vi "Main.vi"(11 "Module Admin":refnum<class "Delacor_lib_QMH_Module Admin.lvclass">) -> ()   [LabVIEW 2020, in "SimpleDependencyInspector.lvlib"]
doc: "This template is based off of the Queued Message Handler design pattern and the Queued Message Handler project template that ships with LabVIEW.\n\nThe main difference is that the queue is private to this module and communication between modules is performed via Broadcast and Request events.\n\nRequest events are wrapped in public API methods and are handled in the Event Handling Loop (EHL) of this VI. Any module can register for Broadcast events sent by this module. The EHL generates messages based on user interface actions.\n\nThe Message Handling Loop (MHL) processes messages generated by the EHL, or by other messages. The messages are string values, so new messages can be added easily to the Message Cases case structure in the MHL. Each message cluster can also provide an optional value for Message Data, which is a variant that can be converted to whatever message-specific data is required.\n_____\nBased on DQMH Project Template 7.0.1.1316.\n\n<b>Note:</b> This VI was modified by the <b>Validate DQMH Module</b> tool to wrap the FP.Open method in the module close code with a Conditional Disable Structure so it does not execute when the Main VI is running as a built EXE."
uses:
  SimpleDependencyInspector.lvlib
  <vilib>/Delacor/Delacor QMH/Libraries/Module Admin_class/Delacor_lib_QMH_Module Admin.lvclass
  Module Data--cluster.ctl
  <vilib>/Delacor/Delacor QMH/Libraries/Message Queue_class/Delacor_lib_QMH_Message Queue.lvclass/Delacor_lib_QMH_Message Queue.ctl
  Stop Argument--cluster.ctl
  Inspect Project Dependencies Argument--cluster.ctl
  Image Type--enum.ctl
  <vilib>/Delacor/Delacor QMH/Libraries/Module Admin_class/Delacor_lib_QMH_Module Admin.lvclass/Delacor_lib_QMH_Module Admin.ctl
  <vilib>/Delacor/Delacor QMH/Libraries/Message Queue_class/Delacor_lib_QMH_Enqueue Message (Single).vi
  <vilib>/Delacor/Delacor QMH/Libraries/Module Admin_class/Delacor_lib_QMH_Get External Launch.vi
  <vilib>/Delacor/Delacor QMH/Libraries/Message Queue_class/Delacor_lib_QMH_Message Queue.lvclass
panel:
  out "Dependencies Plot":picture
  out "error out":errorcluster
  out "Status":string
  in  "Home":bool
  in  "About":bool
  in  "Zoom In":bool
  in  "Zoom Out":bool
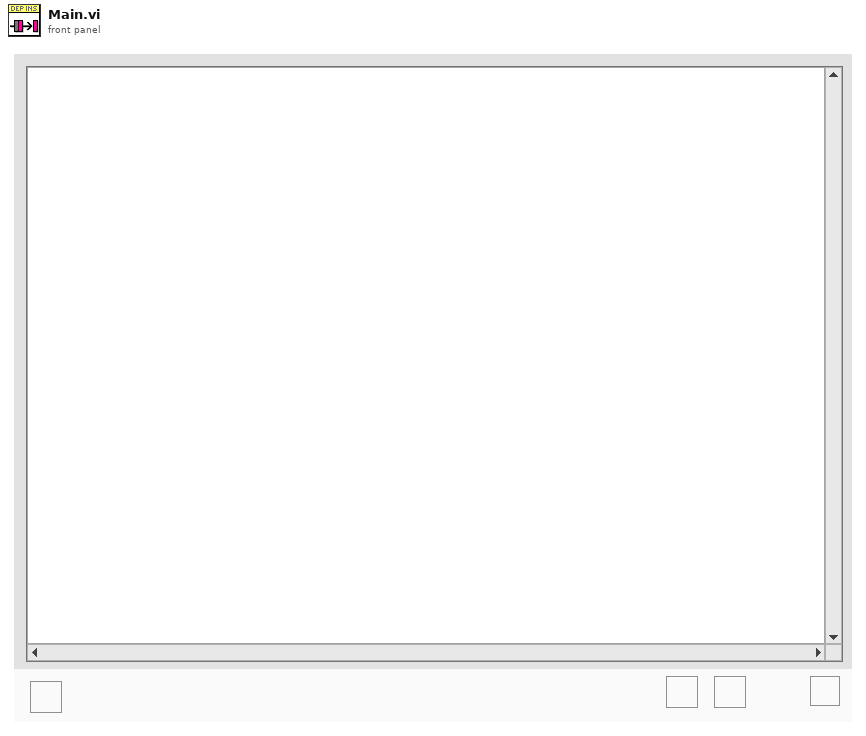
[diagram p1: front panel]
types:
  T1 = typedef "SimpleDependencyInspector.lvlib/Request Events--cluster.ctl" = cluster{"Stop Module":refnum<user-event>, "Show Panel":refnum<user-event>, "Hide Panel":refnum<user-event>, "Get Module Execution Status":refnum<user-event>, "Show Diagram":refnum<user-event>, "Inspect Project Dependencies":refnum<user-event>, "Private":cluster{"Wake Up HL":refnum<user-event>}}
  T2 = typedef "SimpleDependencyInspector.lvlib/Module Data--cluster.ctl" = cluster{"Status":string}
  T3 = enum32{"invalid lock state", "Not Locked", "Locked (No Password)", "Password-protected"}
  T4 = typedef "SimpleDependencyInspector.lvlib/Stop Argument--cluster.ctl" = cluster{"Origin":string, "Exit via Stop Module Req?":bool, "Wait for Module to stop?":bool}
  T5 = typedef "SimpleDependencyInspector.lvlib/Inspect Project Dependencies Argument--cluster.ctl" = cluster{"Path(s) Selection":path[], "Include vi.lib":bool, "pattern Search":string[], "pattern To include in Plot":string[], "Working Path":path, "Img Type":T6}
  T6 = typedef "SimpleDependencyInspector.lvlib/Image Type--enum.ctl" = enum16{"JPEG", "PNG", "BMP", "SVG"}
  T7 = enum32{"Invalid", "Standard", "Closed", "Hidden", "Minimized", "Maximized"}
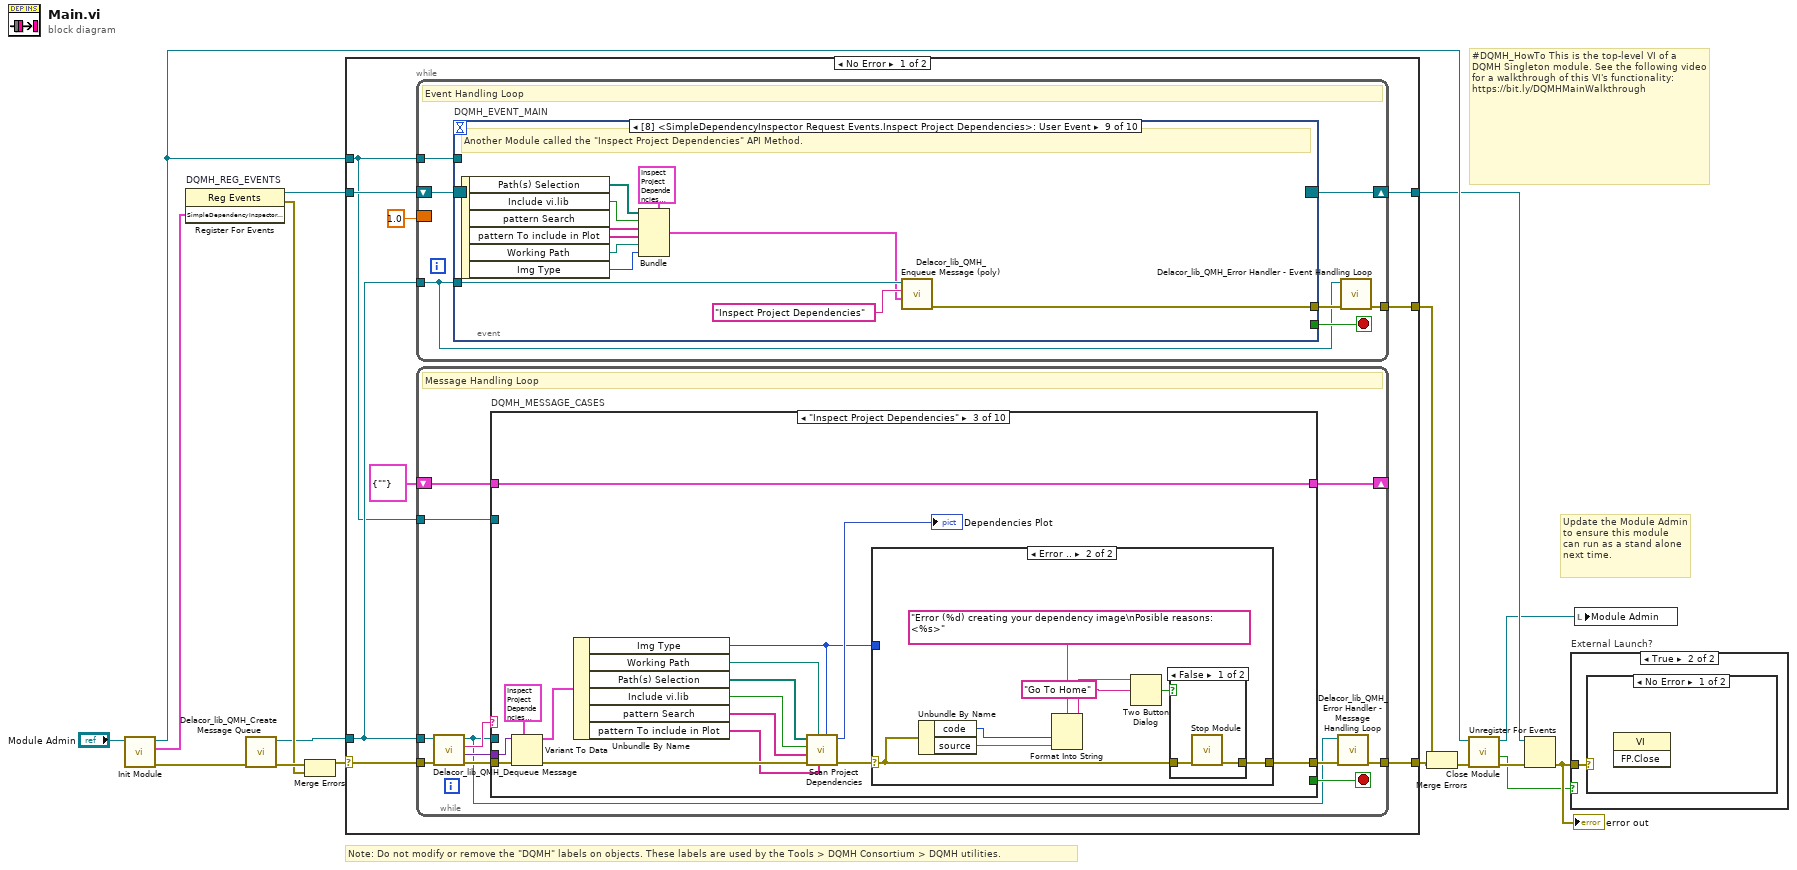
[diagram p0: block diagram]
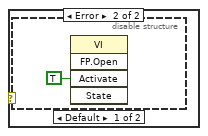
[diagram p3: hidden frame]
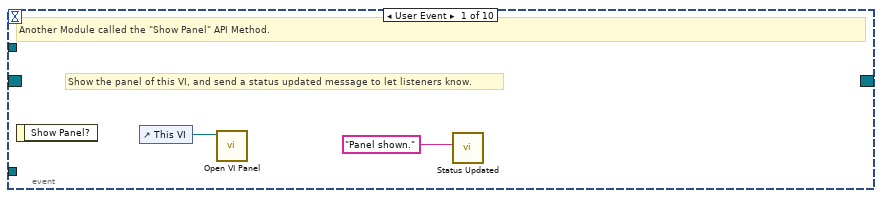
[diagram p5: hidden frame]
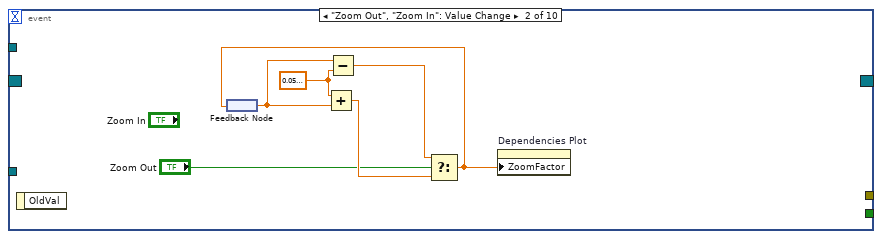
[diagram p6: hidden frame]
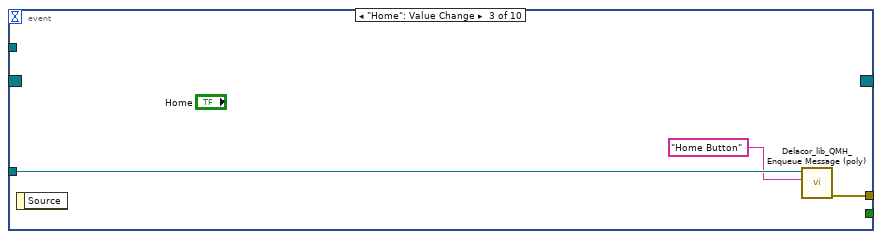
[diagram p7: hidden frame]
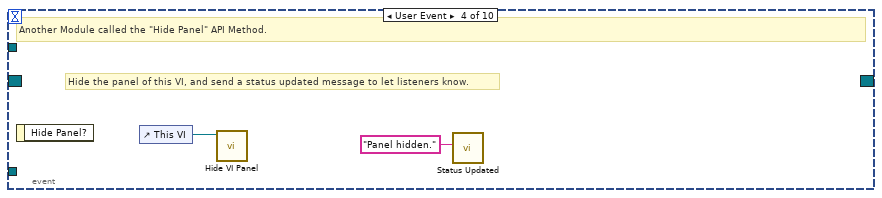
[diagram p8: hidden frame]
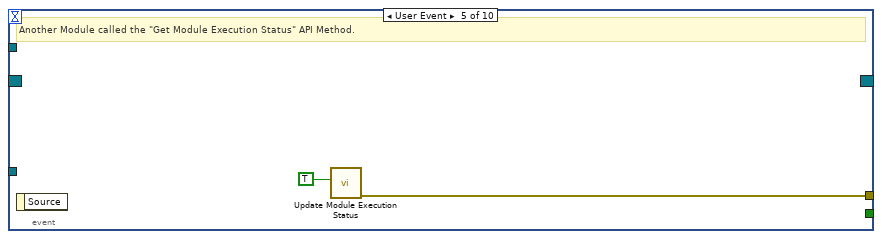
[diagram p9: hidden frame]
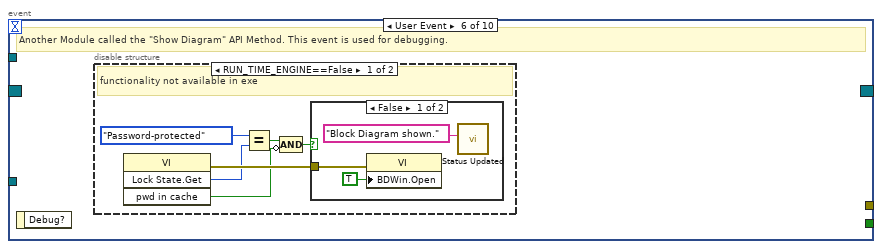
[diagram p10: hidden frame]
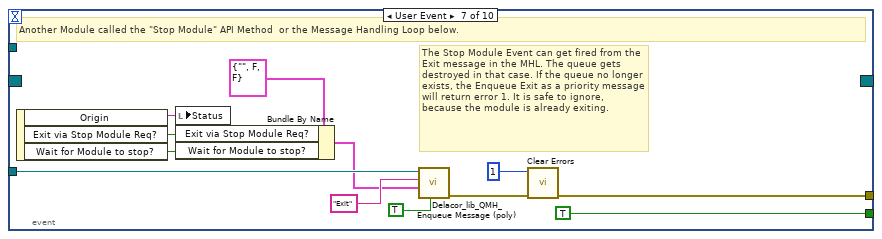
[diagram p13: hidden frame]
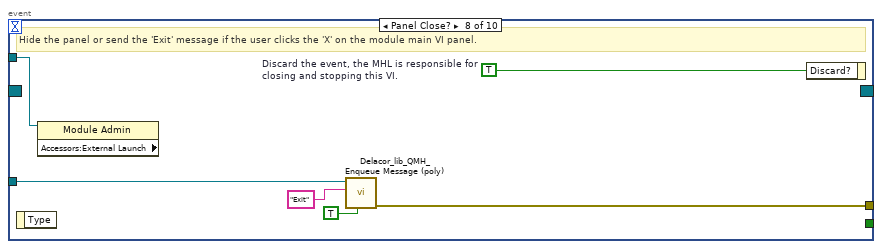
[diagram p14: hidden frame]
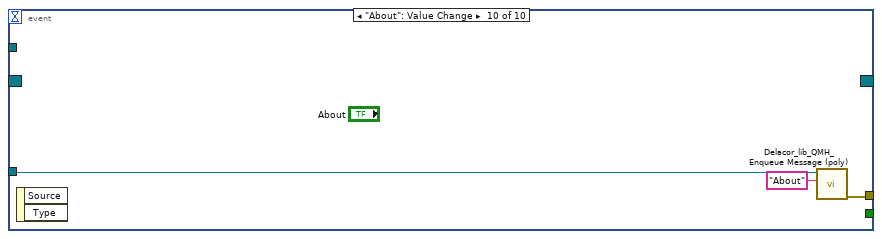
[diagram p15: hidden frame]
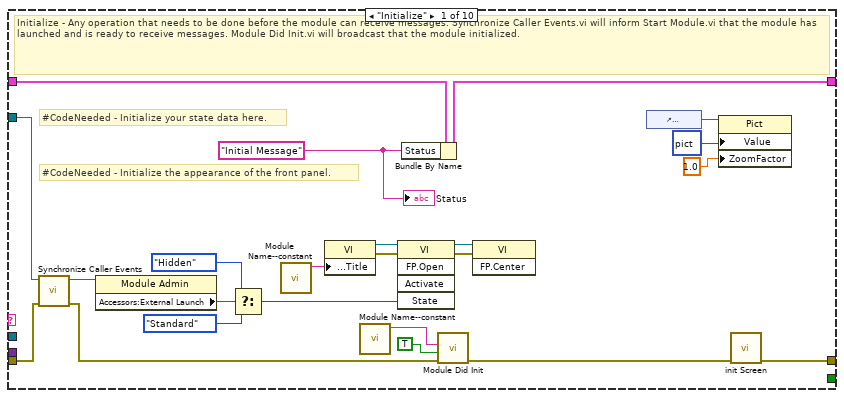
[diagram p16: hidden frame]
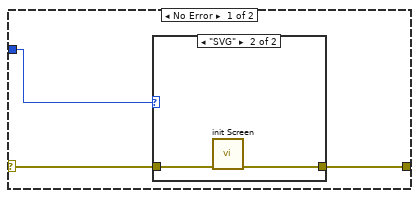
[diagram p18: hidden frame]
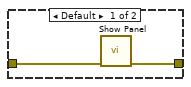
[diagram p19: hidden frame]
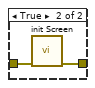
[diagram p20: hidden frame]
diagram:
  # "#DQMH_HowTo This is the top-level VI of a DQMH Singleton module. See the following video for a walkthrough of this VI's functionality: https://bit.ly/DQMHMainWalkthrough"
  # "Note: Do not modify or remove the \"DQMH\" labels on objects. These labels are used by the Tools > DQMH Consortium > DQMH utilities."
  # "Update the Module Admin to ensure this module can run as a stand alone next time."
  n1 = call "Init Module.vi"("Singleton Module Admin in"="Module Admin") -> ("error out"=w16:errorcluster, "SimpleDependencyInspector Request Events"=w1:T1, "Singleton Module Admin out"=w8:refnum<class "Delacor_lib_QMH_Module Admin.lvclass">)  [unwired: 8 in]
  n2 = register-events "DQMH_REG_EVENTS"(w1) -> (reference out=w6:refnum<event-registration>, error out=w9:errorcluster)  [unwired: 2 in]
  n3 = call <vilib>:"Delacor_lib_QMH_Create Message Queue.vi"("error in"=w16) -> ("error out"=w11:errorcluster, "Message Queue"=w5:refnum<class "Delacor_lib_QMH_Message Queue.lvclass">)  [unwired: 9 in]
  n4 = Merge Errors(w11, w9) -> (w10:errorcluster)
  n5 = case shown="No Error" w10 {
    selector: w10 -> [w24 w224]
    tunnel: [w26 w223] -> w17
    tunnel: [w23 w222] -> w7
    tunnel: w6 -> [w21 w222]
    tunnel: w5 -> [w20 w217]
    tunnel: [w25 _] -> w14
    tunnel: w8 -> [w19 w218]
    frame No Error {
      n6 = while {
        tunnel: w20 -> [w27]
        shift-right: [w30] -> w23
        shift-left: w21 -> [w31]
        tunnel: [w32] -> w25
        tunnel: w19 -> [w28]
        border: sgl 1.0 -> [_]
        stop <- w29 stop-if-true
        # "Event Handling Loop"
        n7 = event "DQMH_EVENT_MAIN" shown="[8] <SimpleDependencyInspector Request Events.Inspect Project Dependencies>: User Event" {
          selector: w31 -> [_ _ _ _ _ _ _ _ _ _]
          dyn-events: [_ _ _ _ _ _ _ _ _ _] -> w30
          timeout: _ -> [_ _ _ _ _ _ _ _ _ _]
          tunnel: [_ _ _ _ _ _ TRUE ("Discard?") _ _ _] -> w29
          tunnel: w27 -> [_ _ w43 _ _ _ w65 w73 w85 w88]
          tunnel: [_ _ w44 _ w48 _ w68 w75 w86 w89] -> w33
          tunnel: w28 -> [_ _ _ _ _ _ _ w72 _ _]
          event User Event {
            # "Show the panel of this VI, and send a status updated message to let listeners know."
            # "Another Module called the \"Show Panel\" API Method."
            n8 = event-data() -> ()  [unwired: 1 in, 1 out]
            n9 = control-ref of="This VI"() -> (w35:refnum<vi>)
            n10 = call "Open VI Panel.vi"("VI"=w35) -> ()  [unwired: 10 in, 1 out]
            n11 = call "Status Updated.vi"("Status"="Panel shown." ("format string")) -> ()  [unwired: 10 in, 1 out]
          }
          event "Zoom Out", "Zoom In": Value Change {
            w39 = sgl 0.05 ("x")
            n12 = event-data() -> ()  [unwired: 1 in, 1 out]
            n13 = feedback #1() -> (w40:sgl)
            n14 = Add(x=w39, y=w40) -> (x+y=w38:sgl)
            n15 = Subtract(x=w40, y=w39) -> (x-y=w41:sgl)
            n16 = Select(t=w41, s="Zoom Out", f=w38) -> (s? t:f=w37:sgl)
            n17 = feedback-in #1(w37) -> ()
            n18 = property on="Dependencies Plot" class="Pict"("ZoomFactor"=w37) -> ()  [unwired: 2 in, 2 out]
          }
          event "Home": Value Change {
            n19 = event-data() -> ()  [unwired: 1 in, 1 out]
            n20 = call-poly <vilib>:"Delacor_lib_QMH_Enqueue Message (poly).vi"("Message"="Home Button", "Message Queue in"=w43) -> ("error out"=w44:errorcluster)  [unwired: 8 in, 1 out]
          }
          event User Event {
            # "Hide the panel of this VI, and send a status updated message to let listeners know."
            # "Another Module called the \"Hide Panel\" API Method."
            n21 = event-data() -> ()  [unwired: 1 in, 1 out]
            n22 = control-ref of="This VI"() -> (w46:refnum<vi>)
            n23 = call "Hide VI Panel.vi"("VI"=w46) -> ()  [unwired: 10 in, 1 out]
            n24 = call "Status Updated.vi"("Status"="Panel hidden." ("format string")) -> ()  [unwired: 10 in, 1 out]
          }
          event User Event {
            # "Another Module called the \"Get Module Execution Status\" API Method."
            n25 = event-data() -> ()  [unwired: 1 in, 1 out]
            n26 = call "Update Module Execution Status.vi"("Running?"=TRUE) -> ("error out"=w48:errorcluster)  [unwired: 10 in]
          }
          event User Event {
            # "Another Module called the \"Show Diagram\" API Method. This event is used for debugging."
            n27 = event-data() -> ()  [unwired: 1 in, 1 out]
            n28 = disable-structure shown="RUN_TIME_ENGINE==False" {
              frame condition #0 (active) {
                # "functionality not available in exe"
                n29 = invoke on="Invoke Node" class="VI" method="Lock State.Get"() -> (error out=w54:errorcluster, "Get Lock State"=w53:T3, "pwd in cache"=w50:bool)  [unwired: 4 in, 1 out]
                n30 = Equal?(x=T3."Password-protected", y=w53) -> (x = y?=w51:bool)
                n31 = Compound Arithmetic op=AND(w51, invert w50) -> (w49:bool)
                n32 = case shown="False" w49 {
                  tunnel: w54 -> [w57 _]
                  frame False {
                    n33 = property on="Property Node" class="VI"(error in=w57, "BDWin.Open"=TRUE ("Block Diagram Window:Open")) -> ()  [unwired: 1 in, 2 out]
                    n34 = call "Status Updated.vi"("Status"="Block Diagram shown." ("format string")) -> ()  [unwired: 10 in, 1 out]
                  }
                  frame True {
                    # "Password-protected VI, and the password is not in the cache. Do not show the diagram."
                  }
                }
              }
              frame condition #1 {
              }
            }
          }
          event User Event {
            # "The Stop Module Event can get fired from the Exit message in the MHL. The queue gets destroyed in that case. If the queue no longer exists, the Enqueue Exit as a priority message will return error 1. It is safe to ignore, because the module is already exiting."
            # "Another Module called the \"Stop Module\" API Method  or the Message Handling Loop below."
            n35 = event-data() -> ("Origin"=w64:string, "Exit via Stop Module Req?"=w60:bool, "Wait for Module to stop?"=w59:bool)  [unwired: 1 in]
            n36 = local write "Status"(w64) -> ()
            n37 = Bundle By Name(cluster=T4 {"Origin"="", "Exit via Stop Module Req?"=FALSE, "Wait for Module to stop?"=FALSE} ("Stop Argument"), "Exit via Stop Module Req?"=w60, "Wait for Module to stop?"=w59) -> (w58:T4)
            n38 = call-poly <vilib>:"Delacor_lib_QMH_Enqueue Message (poly).vi"("Priority Message? (F)"=TRUE, "Message Data"=w58, "Message"="Exit", "Message Queue in"=w65) -> ("error out"=w69:errorcluster)  [unwired: 6 in, 1 out]
            n39 = call <vilib>:"Clear Errors.vi"("error in (no error)"=w69, "specific error code to clear (0: all)"=1) -> ("error out"=w68:errorcluster)  [unwired: 4 in, 1 out]
          }
          event Panel Close? {
            w74 = TRUE  # Discard the event, the MHL is responsible for closing and stopping this VI.
            # "Hide the panel or send the 'Exit' message if the user clicks the 'X' on the module main VI panel."
            n40 = event-data() -> ()  [unwired: 1 in, 1 out]
            n41 = property on="Property Node" class="Module Admin" props=["Accessors:External Launch"](reference=w72) -> ()  [unwired: 1 in, 3 out]
            n42 = call-poly <vilib>:"Delacor_lib_QMH_Enqueue Message (poly).vi"("Priority Message? (F)"=TRUE, "Message"="Exit", "Message Queue in"=w73) -> ("error out"=w75:errorcluster)  [unwired: 7 in, 1 out]
            n43 = event-data ("Event Filter Node")("Discard?"=w74) -> ()  [unwired: 1 in, 1 out]
          }
          event User Event {
            # "Another Module called the \"Inspect Project Dependencies\" API Method."
            n44 = event-data() -> ("Path(s) Selection"=w81:path[], "Include vi.lib"=w80:bool, "pattern Search"=w79:string[], "pattern To include in Plot"=w78:string[], "Working Path"=w77:path, "Img Type"=w76:T6)  [unwired: 1 in]
            n45 = Bundle(cluster=T5 {"Path(s) Selection"=[], "Include vi.lib"=FALSE, "pattern Search"=["*.lvlib", "*.lvclass"], "pattern To include in Plot"=["*.lvlib", "*.lvclass"], "Working Path"=path "", "Img Type"=enum."JPEG"} ("Inspect Project Dependencies Argument"), "Path(s) Selection"=w81, "Include vi.lib"=w80, "pattern Search"=w79, "pattern To include in Plot"=w78, "Working Path"=w77, "Img Type"=w76) -> (w82:T5)
            n46 = call-poly <vilib>:"Delacor_lib_QMH_Enqueue Message (poly).vi"("Message Data"=w82, "Message"="Inspect Project Dependencies", "Message Queue in"=w85) -> ("error out"=w86:errorcluster)  [unwired: 7 in, 1 out]
          }
          event "About": Value Change {
            n47 = event-data() -> ()  [unwired: 1 in, 2 out]
            n48 = call-poly <vilib>:"Delacor_lib_QMH_Enqueue Message (poly).vi"("Message"="About", "Message Queue in"=w88) -> ("error out"=w89:errorcluster)  [unwired: 8 in, 1 out]
          }
        }
        n49 = call-dynamic "Delacor_lib_QMH_Error Handler - Event Handling Loop.vi"("error in"=w33, "Message Queue in"=w27) -> ("dup error in"=w32:errorcluster)  [unwired: 8 in, 1 out]
      }
      n50 = while {
        tunnel: w20 -> [w90]
        shift-right: [w96] -> _
        shift-left: T2 {"Status"=""} ("Data Cluster") -> [w97]
        tunnel: w24 -> [w101]
        tunnel: [w99] -> w26
        tunnel: w19 -> [w92]
        stop <- w95 stop-if-true
        # "Message Handling Loop"
        n51 = call-dynamic "Delacor_lib_QMH_Dequeue Message.vi"("error in"=w101, "Message Queue in"=w90) -> ("error out"=w100:errorcluster, "Message Data"=w93:variant, "Message"=w94:string, "Message Queue out"=w91:refnum<class "Delacor_lib_QMH_Message Queue.lvclass">)  [unwired: 6 in]
        n52 = case "DQMH_MESSAGE_CASES" shown="\"Inspect Project Dependencies\"" w94 {
          selector: w94 -> [_ _ _ _ _ _ _ _ _ w212]
          tunnel: w91 -> [_ _ _ _ _ _ _ w177 w200 _]
          tunnel: w100 -> [w122 w126 w141 w164 w169 w172 w174 w185 w206 w215]
          tunnel: [w119 w126 w138 w162 w166 w171 w174 w181 w201 w216] -> w98
          tunnel: w97 -> [w110 w125 w137 w161 w165 w170 w173 w179 w199 w213]
          tunnel: [w109 w125 w137 w161 w165 w170 w173 w179 w199 w213] -> w96
          tunnel: [_ _ _ _ _ _ _ _ w198 _] -> w95
          tunnel: w93 -> [_ _ w136 _ _ _ _ w178 w197 _]
          tunnel: w92 -> [w111 _ _ _ _ _ _ w176 w192 _]
          frame "Initialize" {
            w105 = "Initial Message" ("Initial Message")
            # "#CodeNeeded - Initialize the appearance of the front panel."
            # "#CodeNeeded - Initialize your state data here."
            # "Initialize - Any operation that needs to be done before the module can receive messages. Synchronize Caller Events.vi will inform Start Module.vi that the module has launched and is ready to receive messages. Module Did Init.vi will broadcast that the module initialized."
            n53 = call "Synchronize Caller Events.vi"("error in"=w122, "Singleton Module Admin in"=w111) -> ("error out"=w121:errorcluster, "Singleton Module Admin out"=w106:refnum<class "Delacor_lib_QMH_Module Admin.lvclass">)  [unwired: 8 in]
            n54 = property on="Property Node" class="Module Admin"(reference=w106) -> ("Accessors:External Launch"=w115:bool)  [unwired: 1 in, 2 out]
            n55 = Select(t=T7."Hidden" ("State"), s=w115, f=T7."Standard" ("State")) -> (s? t:f=w112:T7)
            n56 = call "Module Name--constant.vi"() -> ("Module Name"=w118:string)  [unwired: 11 in]
            n57 = property on="Property Node" class="VI"("Front Panel.Title"=w118) -> (reference out=w117:refnum<vi>, error out=w124:errorcluster)  [unwired: 2 in]
            n58 = call "Module Name--constant.vi"() -> ("Module Name"=w107:string)  [unwired: 11 in]
            n59 = invoke on="Invoke Node" class="VI" method="FP.Open"(reference=w117, error in=w124, "State"=w112) -> (reference out=w116:refnum<vi>, error out=w123:errorcluster)  [unwired: 2 in, 3 out]
            n60 = Bundle By Name(cluster=w110, "Status"=w105) -> (w109:T2)
            n61 = call "Module Did Init.vi"("error in"=w121, "Initialized?"=TRUE, "Origin"=w107) -> ("error out"=w120:errorcluster)  [unwired: 8 in]
            n62 = invoke on="Invoke Node" class="VI" method="FP.Center"(reference=w116, error in=w123) -> ()  [unwired: 1 in, 3 out]
            n63 = control-ref of="Dependencies Plot"() -> (w103:refnum<vi>)
            n64 = property class="Pict"(reference=w103, "Value"=picture data[5B], "ZoomFactor"=sgl 1.0 ("Zoom Factor")) -> ()  [unwired: 1 in, 2 out]
            n65 = call "init Screen.vi"("error in"=w120) -> ("error out"=w119:errorcluster)  [unwired: 10 in]
            "Status" <- w105
          }
          frame "---Module Specific---" {
            # "Separator -- The following cases handle messages specific to this Module."
          }
          frame "Inspect Project Dependencies" {
            n66 = Variant To Data(error in=w141, type=T5 {"Path(s) Selection"=[], "Include vi.lib"=FALSE, "pattern Search"=["*.lvlib", "*.lvclass"], "pattern To include in Plot"=["*.lvlib", "*.lvclass"], "Working Path"=path "", "Img Type"=enum."JPEG"} ("Inspect Project Dependencies Argument"), Variant=w136) -> (data=w134:T5, error out=w140:errorcluster)
            n67 = Unbundle By Name(w134) -> ("Img Type"=w127:T6, "Working Path"=w128:path, "Path(s) Selection"=w133:path[], "Include vi.lib"=w132:bool, "pattern Search"=w131:string[], "pattern To include in Plot"=w130:string[])
            n68 = call "Scan Project Dependencies.vi"("Img Type"=w127, "pattern to Include no *"=w130, "Working Path"=w128, "error in"=w140, "pattern Search"=w131, "Include vi.lib"=w132, "Selection"=w133) -> ("error out"=w139:errorcluster, "Dependency Plot"=→"Dependencies Plot":picture)  [unwired: 1 in, 2 out]
            n69 = case shown="Error .." w139 {
              selector: w139 -> [w143 w155]
              tunnel: [w144 w156] -> w138
              tunnel: w127 -> [w142 _]
              frame No Error {
                n70 = case shown="\"SVG\"" w142 {
                  tunnel: [w146 w147] -> w144
                  tunnel: w143 -> [w145 w148]
                  frame Default {
                    n71 = call "Show Panel.vi"("error in"=w145) -> ("error out"=w146:errorcluster)  [unwired: 10 in]
                  }
                  frame "SVG" {
                    n72 = call "init Screen.vi"("error in"=w148) -> ("error out"=w147:errorcluster)  [unwired: 10 in]
                  }
                }
              }
              frame Error {
                n73 = Unbundle By Name(w155) -> ("code"=w150:i32, "source"=w149:string)
                n74 = Format Into String(format string="Error (%d) creating your dependency image\nPosible reasons: <%s>" ("message"), w150, w149) -> (resulting string=w151:string)  [unwired: 2 in, 1 out]
                n75 = Two Button Dialog(message=w151, 2:"Go To Home" ("T button name (\"OK\")")) -> (T button?=w154:bool)  [unwired: 1 in]
                n76 = case shown="False" w154 {
                  tunnel: w155 -> [w158 w160]
                  tunnel: [w157 w159] -> w156
                  frame False {
                    n77 = call "Stop Module.vi"("error in"=w158) -> ("error out"=w157:errorcluster)  [unwired: 10 in]
                  }
                  frame True {
                    n78 = call "init Screen.vi"("error in"=w160) -> ("error out"=w159:errorcluster)  [unwired: 10 in]
                  }
                }
              }
            }
          }
          frame "Home Button" {
            # "User presed Home Button, go to init screen"
            n79 = call "Hide Panel.vi"("error in"=w164) -> ("error out"=w163:errorcluster)  [unwired: 10 in]
            n80 = call "init Screen.vi"("error in"=w163) -> ("error out"=w162:errorcluster)  [unwired: 10 in]
          }
          frame "About" {
            # "User presed Abput Button, go to about screen"
            n81 = call "Hide Panel.vi"("error in"=w169) -> ("error out"=w168:errorcluster)  [unwired: 10 in]
            n82 = call "About Dependency Inspector.vi"("error in"=w168) -> ("error out"=w167:errorcluster)  [unwired: 10 in]
            n83 = call "Show Panel.vi"("error in"=w167) -> ("error out"=w166:errorcluster)  [unwired: 10 in]
          }
          frame "---Copy This Frame---" {
            # "Duplicate this frame when creating new messages.  Change this comment in the duplicated frame to describe this message."
            n84 = Merge Errors(w172) -> (w171:errorcluster)
          }
          frame "---Exit and Error Handling---" {
            # "Separator - The following cases handle errors and exit messages."
          }
          frame "Error" {
            # "#CodeRecommended - If the module is running in standalone mode (External Launch = FALSE), this code will pop up an error dialog and call the 'Exit' message if an error occurs. Add more fine-grained error management here."
            # "Error - Check the error message data and respond accordingly. This message is sent by the \"Error Handler\" VIs at the end of each loop in this application."
            n85 = property on="Property Node" class="Module Admin"(reference=w176) -> ("Accessors:External Launch"=w175:bool)  [unwired: 1 in, 2 out]
            n86 = Variant To Data(error in=w185, type=errorcluster {"status"=FALSE, "code"=0, "source"=""} ("error constant"), Variant=w178) -> (data=w180:errorcluster, error out=w183:errorcluster)
            n87 = local write "error out"(w180) -> ()
            n88 = call "Error Reported.vi"("Error"=w180) -> ()  [unwired: 10 in, 1 out]
            n89 = case shown="True" w175 {
              tunnel: [w190 _] -> w182
              tunnel: w177 -> [w188 _]
              tunnel: w180 -> [w189 _]
              frame False {
                n90 = disable-structure shown="Default" {
                  disable-tunnel: w189 -> [w191 _]
                  frame condition #0 (active) {
                    # "If the module is running standalone, then pop up an error dialog and call the \"Exit\" message."
                    n91 = call <vilib>:"Simple Error Handler.vi"("error in (no error)"=w191) -> ()  [unwired: 4 in, 5 out]
                  }
                  frame condition #1 {
                    # "To prevent the Simple Error Handler VI from being loaded (e.g. when deploying to a Real-Time target), add the Conditional Disable Symbol \"DQMH_Disable_SEH\" to your project and set it to TRUE."
                  }
                }
                n92 = call-poly <vilib>:"Delacor_lib_QMH_Enqueue Message (poly).vi"("Priority Message? (F)"=TRUE, "Message"="Exit", "Message Queue in"=w188) -> ("error out"=w190:errorcluster)  [unwired: 7 in, 1 out]
              }
              frame True {
                # "If the module was launched externally, calling the Error Reported broadcast VI is the only action performed by the \"Error\" message. The module's caller can then process the error appropriately."
              }
            }
            n93 = Merge Errors(w183, w182) -> (w181:errorcluster)
          }
          frame "Exit" {
            w196 = 91  # 91: not all Exit messages will have an argument
            w198 = TRUE  # Stop the VI
            # "Release the message queue reference"
            # "#CodeNeeded - Add any required cleanup code here."
            # "Exit - Exit the application."
            n94 = Variant To Data(error in=w206, type=T4 {"Origin"="", "Exit via Stop Module Req?"=FALSE, "Wait for Module to stop?"=FALSE} ("Stop Argument"), Variant=w197) -> (data=w194:T4, error out=w203:errorcluster)
            n95 = call <vilib>:"Clear Errors.vi"("error in (no error)"=w203, "specific error code to clear (0: all)"=w196) -> ("error out"=w205:errorcluster)  [unwired: 4 in, 1 out]
            n96 = control-ref of="This VI"() -> (w193:refnum<vi>)
            n97 = call-dynamic "Delacor_lib_QMH_Release Message Queue.vi"("error in"=w205, "Message Queue"=w200) -> ("error out"=w204:errorcluster)  [unwired: 9 in]
            n98 = call "Handle Exit.vi"("Stop Argument"=w194, "Admin in"=w192, "VI reference"=w193) -> ("error out"=w202:errorcluster)  [unwired: 7 in, 1 out]
            n99 = Merge Errors(w204, w202) -> (w201:errorcluster)
            n100 = call "Error Reported.vi"("Error"=w201) -> ()  [unwired: 10 in, 1 out]
          }
          frame Default {
            # "'Default' case only runs if there is a message that isn't defined in any of the other cases.  Output a programming error."
            n101 = call "Module Name--constant.vi"() -> ("Module Name"=w211:string)  [unwired: 11 in]
            n102 = Format Into String(format string="The invalid message string \"%s\" was received in the Message Handling Loop for module \"%s\".", w212, w211) -> (resulting string=w207:string)  [unwired: 2 in, 1 out]
            n103 = call <vilib>:"Error Cluster From Error Code.vi"("show call chain? (False)"=TRUE, "error message (\"\")"=w207, "error code (0)"=1) -> ("error out"=w214:errorcluster)  [unwired: 6 in]
            n104 = Merge Errors(w215, w214) -> (w216:errorcluster)
          }
        }
        n105 = call-dynamic "Delacor_lib_QMH_Error Handler - Message Handling Loop.vi"("error in"=w98, "Message Queue in"=w91) -> ("dup error in"=w99:errorcluster)  [unwired: 8 in, 1 out]
      }
    }
    frame Error {
      # "Synchronize Caller Events.vi will inform Start Module.vi that the module has launched and will let the code calling Start Module.vi register for broadcasts and would permit the caller receive the broadcast that an error occurred at launch time."
      n106 = call-dynamic "Delacor_lib_QMH_Release Message Queue.vi"("error in"=w224, "Message Queue"=w217) -> ("error out"=w223:errorcluster)  [unwired: 9 in]
      n107 = call "Synchronize Caller Events.vi"("Singleton Module Admin in"=w218) -> ("error out"=w225:errorcluster)  [unwired: 9 in, 1 out]
      n108 = call "Module Name--constant.vi"() -> ("Module Name"=w221:string)  [unwired: 11 in]
      n109 = Format Into String(format string="An error occurred during initialization. %s is no longer running.", w221) -> (resulting string=w219:string)  [unwired: 2 in, 1 out]
      n110 = Merge Errors(w223, w225) -> (w226:errorcluster)
      n111 = call "Error Reported.vi"("Additional Information"=w219, "Error"=w226) -> ()  [unwired: 9 in, 1 out]
    }
  }
  n112 = Merge Errors(w14, w17) -> (w13:errorcluster)
  n113 = call "Close Module.vi"("error in"=w13, "Module Admin in"=w8) -> ("error out"=w15:errorcluster, "External Launch"=w2:bool, "Module Admin out"=w3:refnum<class "Delacor_lib_QMH_Module Admin.lvclass">)  [unwired: 7 in]
  n114 = Unregister For Events(event registration refnum=w7, error in=w15) -> (error out=w12:errorcluster)
  "error out" <- w12
  n115 = case "External Launch?" shown="True" w2 {
    tunnel: w12 -> [_ w227]
    frame False {
    }
    frame True {
      n116 = case shown="No Error" w227 {
        frame No Error {
          n117 = invoke on="Invoke Node" class="VI" method="FP.Close"() -> ()  [unwired: 3 in, 3 out]
        }
        frame Error {
          n118 = disable-structure shown="Default" {
            frame condition #0 (active) {
              n119 = invoke class="VI" method="FP.Open"("Activate"=TRUE ("Activate?")) -> ()  [unwired: 4 in, 5 out]
            }
            frame condition #1 {
              # "Don't show panel on error if running inside a built EXE."
            }
          }
        }
      }
    }
  }
  n120 = local write "Module Admin"(w3) -> ()
